vi "Get VISA Session.vi"(8 "error in":errorcluster, 11 "Scope VISA in":refnum<class "Scope VISA.lvclass">) -> (0 "error out":errorcluster, 2 "VISA session":refnum<visa-resource-name>, 3 "Scope VISA out":refnum<class "Scope VISA.lvclass">)   [LabVIEW 2023, in "Scope.lvlib" / "Scope VISA.lvlib" / "Scope VISA.lvclass"]
uses:
  Scope VISA.lvclass
  Scope Base/Scope Base.lvclass/Scope Base.ctl
  Configuration/Scope VISA CFG.lvclass
  Configuration/Scope VISA CFG.lvclass/Scope VISA CFG.ctl
  Scope VISA.lvclass/Scope VISA.ctl
  Scope Base/Scope Base.lvclass
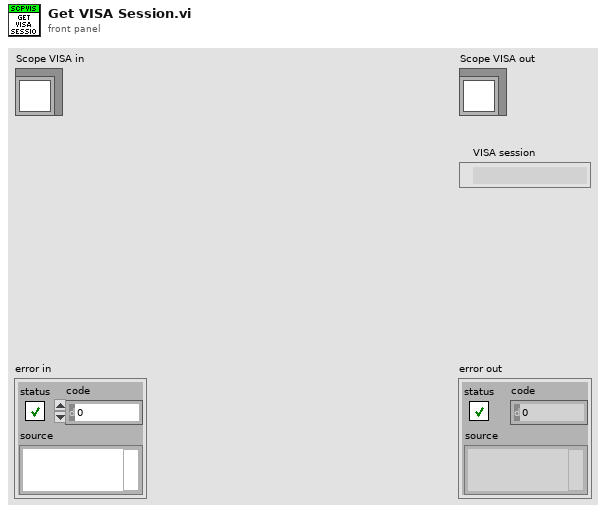
[diagram p1: front panel]
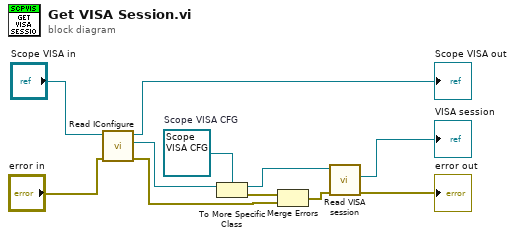
[diagram p0: block diagram]
diagram:
  w8 = refnum<class "Scope VISA CFG.lvclass"> refnum  # Scope VISA CFG
  n1 = call "Read IConfigure.vi"("error in (no error)"="error in", "Scope Base in"="Scope VISA in") -> ("error out"=w1:errorcluster, "IConfigureScope"=w9:refnum<class "IConfigure.lvclass">, "Scope Base out"=→"Scope VISA out":refnum<class "Scope VISA.lvclass">)  [unwired: 7 in]
  n2 = To More Specific Class(target class=w8, reference=w9) -> (specific class reference=w5:refnum<class "Scope VISA CFG.lvclass">, error out=w7:errorcluster)  [unwired: 1 in]
  n3 = Merge Errors(w7, w1) -> (w2:errorcluster)
  n4 = call "Read VISA session.vi"("error in (no error)"=w2, "Scope VISA CFG in"=w5) -> ("error out"=→"error out":errorcluster, "VISA session"=→"VISA session":refnum<visa-resource-name>)  [unwired: 7 in, 1 out]
